vi "cblas ddot.vi"(5 "n":i32=-1, 6 "incy":i32=1, 7 "incx":i32=1, 10 "y":dbl[](array[numeric]), 11 "x":dbl[](array[numeric])) -> (0 "error":i32, 3 "ddot":dbl)   [LabVIEW 2014, in "NI_AALBLAS.lvlib"]
uses:
  NI_AALBLAS.lvlib
  lvblas.dll
panel:
  # "double cblas_ddot(n, *x, incx, *y, incy)"
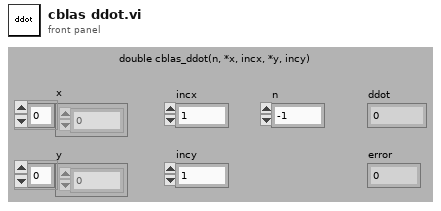
[diagram p1: front panel]
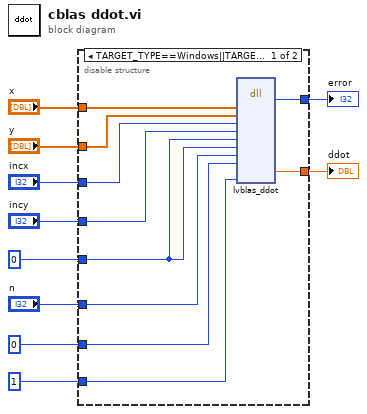
[diagram p0: block diagram]
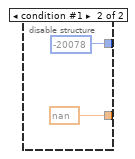
[diagram p2: hidden frame]
diagram:
  n1 = disable-structure shown="TARGET_TYPE==Windows||TARGET_TYPE==Unix||TARGET_TYPE==RT||TARGET_TYPE==Mac" {
    disable-tunnel: [w20 nan] -> w10
    disable-tunnel: "x" -> [w19 _]
    disable-tunnel: "y" -> [w18 _]
    disable-tunnel: "n" -> [w17 _]
    disable-tunnel: [w16 -20078] -> w6
    disable-tunnel: 0 -> [w15 _]
    disable-tunnel: 0 ("OpX") -> [w14 _]
    disable-tunnel: "incx" -> [w13 _]
    disable-tunnel: "incy" -> [w12 _]
    disable-tunnel: 1 ("OpX") -> [w11 _]
    frame condition #0 (active) {
      n2 = dll-call lib="C:/Program Files (x86)/National Instruments/LabVIEW 2014/resource/lvblas.*" fn="lvblas_ddot" ("CBLAS.dll:DotProdH")("X"=w19, "Y"=w18, "IncX"=w13, "IncY"=w12, "startX"=w15, "startY"=w15, "N"=w17, "OpX"=w14, "check"=w11) -> ("error"=w16:i32, "DotProd"=w20:dbl)  [unwired: 12 in, 3 out]
    }
    frame condition #1 {
    }
  }
  "error" <- w6
  "ddot" <- w10
